vi "setUp.vi"(8 "error in (no error)":errorcluster, 11 "reference in":refnum<class "WaitOnTestComplete.lvclass">) -> (0 "error out":errorcluster, 3 "reference in":refnum<class "WaitOnTestComplete.lvclass">)   [LabVIEW 2013, in "WaitOnTestComplete.lvclass"]
uses:
  WaitOnTestComplete.lvclass
  WaitOnTestComplete.lvclass/WaitOnTestComplete.ctl
  Classes/TestCase/TestCase.lvclass
panel:
  # "Copyright © 2007 James Kring, Inc. All rights reserved.\n\nAuthor: Jim Kring [jim.kring@jameskring.com]\n\nThis library is provided \"AS IS\" ,WITHOUT WARRANTIES OR \nCONDITIONS OF ANY KIND, either express or implied.\n\nJames Kring, Inc. -- http://www.jameskring.com"
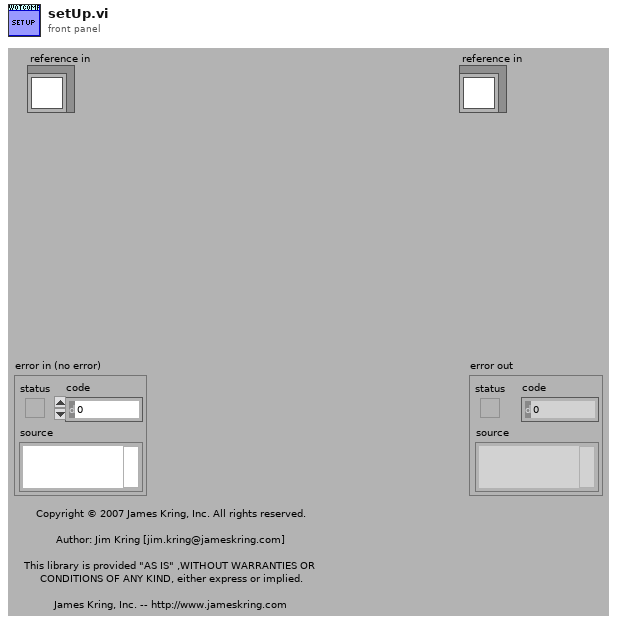
[diagram p1: front panel]
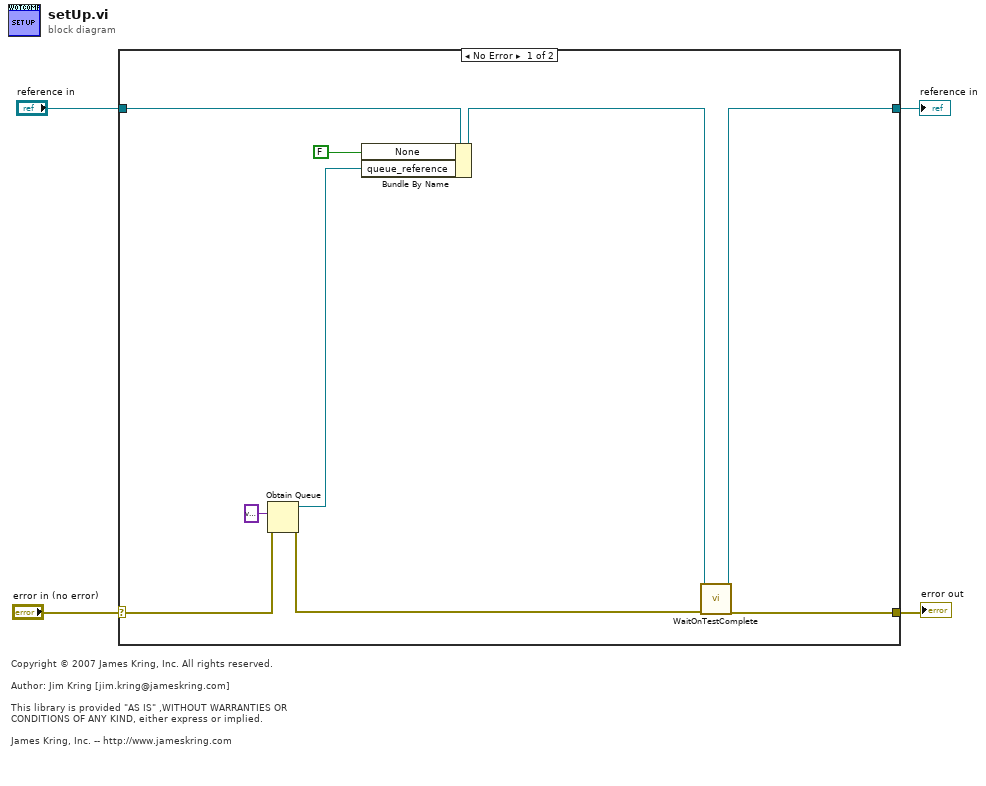
[diagram p0: block diagram]
diagram:
  # "Copyright © 2007 James Kring, Inc. All rights reserved.\n\nAuthor: Jim Kring [jim.kring@jameskring.com]\n\nThis library is provided \"AS IS\" ,WITHOUT WARRANTIES OR \nCONDITIONS OF ANY KIND, either express or implied.\n\nJames Kring, Inc. -- http://www.jameskring.com"
  n1 = case shown="No Error" "error in (no error)" {
    selector: "error in (no error)" -> [w7 w15]
    tunnel: [w10 w15] -> w3
    tunnel: [w11 w14] -> w1
    tunnel: "reference in" -> [w13 w14]
    frame No Error {
      n2 = Obtain Queue(element data type=variant, error in (no error)=w7) -> (queue out=w8:refnum<queue>, error out=w5:errorcluster)  [unwired: 3 in, 1 out]
      n3 = Bundle By Name(cluster=w13, "None"=FALSE, "queue_reference"=w8) -> (w6:refnum<class "WaitOnTestComplete.lvclass">)
      n4 = call "WaitOnTestComplete.vi"("error in (no error)"=w5, "TestCase in"=w6) -> ("error out"=w10:errorcluster, "TestCase out"=w11:refnum<class "WaitOnTestComplete.lvclass">)  [unwired: 8 in]
    }
    frame Error {
    }
  }
  "error out" <- w3
  "reference in" <- w1
